vi "ROI entry screen-LBox edit cells.vi"(8 "error in (no error)":errorcluster, 11 "Selected Cell":T1) -> (0 "error out":errorcluster)   [LabVIEW 2020]
uses:
  <vilib>/Utility/miscctls.llb/LVRowAndColumnTypeDef.ctl
  Typedefs/ROI management FG states.ctl
  Typedefs/ROI Variable resolution info.ctl
  Typedefs/FGV ROI Time Ops.ctl
  Globals/gl_ROI Entry UI globals.vi
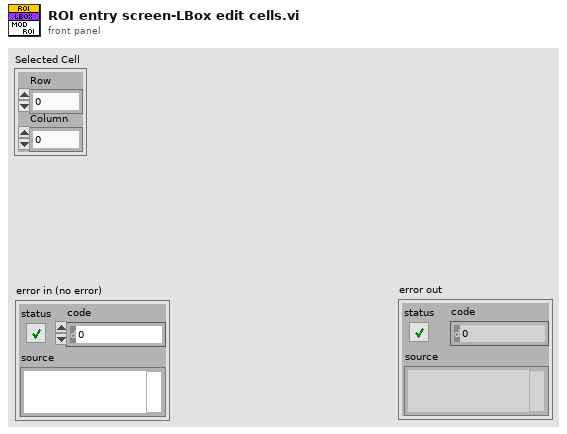
[diagram p1: front panel]
types:
  T1 = typedef "LVRowAndColumnTypeDef.ctl" = cluster{"Row":i32, "Column":i32}
  T2 = typedef "ROI management FG states.ctl" = enum16{"Read", "Write", "Write-from dataset", "Clear Last", "Clear All", "Delete ROI", "Update ROIs time", "Reload last ROI set", "Modify ROI Parameters", "Offset all ROI", "Offset visible ROI", "Modify Dwell Time", "Modify Laser Power"}
  T3 = typedef "ROI entry screen ctrl refs cluster.ctl" = cluster{"Done button":refnum<vi>, "Imaging button":refnum<vi>, "Acquisition button":refnum<vi>, "Scan dwell time per pixel (us)":refnum<vi>, "# of planes":refnum<vi>, "Zoom Ctrl":refnum<vi>, "Equal size":refnum<vi>, "Channel":refnum<vi>, "Image Display":refnum<vi>, "Z-Plane Selector":refnum<vi>, "Number of lines left":refnum<vi>, "Z-stack folder path":refnum<vi>, "POI Density":refnum<vi>, "Arb Plane Entry":refnum<vi>, "Whole Plane":refnum<vi>, "Line Mode":refnum<vi>, "Clear Last":refnum<vi>, "Clear All":refnum<vi>, "Delete Lines":refnum<vi>, "Trial Length (sec)":refnum<vi>, "Palette Type":refnum<vi>, "Intensity slider":refnum<vi>, "# POI":refnum<vi>, "Max Z Proj":refnum<vi>, "Zplane ind":refnum<vi>, "Wavelength (nm)":refnum<vi>, "Number of Trials":refnum<vi>, "Funct stim.trig.enable":refnum<vi>, "Funct stim.trig.delay (s)":refnum<vi>, "Line Mode":refnum<vi>, "Step size (µm)":refnum<vi>, "ROI move mode":refnum<vi>, "Cool-down time (s)":refnum<vi>, "Enable cool-down time":refnum<vi>, "Motor Z ind. (um)":refnum<vi>, "AOL Z ind. (um)":refnum<vi>, "Load Reference Image":refnum<vi>, "Rel.  Res.":refnum<vi>, "ROI LIST":refnum<vi>, "Show All":refnum<vi>, "ROI Type":refnum<vi>, "Start Plane":refnum<vi>, "Stop Plane":refnum<vi>, "Offset ROI":refnum<vi>, "Tab Control":refnum<vi>, "Laser Power(%)":refnum<vi>, "Cycle rate":refnum<vi>, "FOV (Ind.)":refnum<vi>, "Frame Size (Ind.)":refnum<vi>, "Resolution (Ind.)":refnum<vi>, "Pixel Density (Ind)":refnum<vi>, "Laser Power (Ind.)":refnum<vi>, "Dwell Time (Ind.)":refnum<vi>, "Adj MC":refnum<vi>}
  T4 = typedef "ROI parameters data type.ctl" = cluster{"ROI index":dbl, "ROI ID":dbl, "ROI Time (ns)":dbl, "Pixels in ROI":dbl, "X start":dbl, "Y start":dbl, "Z start":dbl, "X stop":dbl, "Y stop":dbl, "Z stop":dbl, "Angle (deg)":dbl, "Composite ID":dbl, "Number of lines":dbl, "Frame Size":dbl, "Zoom":dbl, "Laser Power (%)":dbl, "ROI group ID":dbl, "Resolution":dbl, "Dwell Time per pixel":dbl, "Pixels per miniscan":dbl, "Original FOV (um)":dbl, "Apparent Frame Size":dbl, "Z Plane Idx":i32[], "Z Plane codes":i32[]}
  T5 = typedef "ROI Variable resolution info.ctl" = cluster{"Resolution":dbl, "Pixel Density":dbl, "Relative Resolution":dbl, "Apparent frame size":dbl}
  T6 = typedef "FGV ROI Time Ops.ctl" = enum16{"Read", "Write Cycle Time", "Write Cycle Rate"}
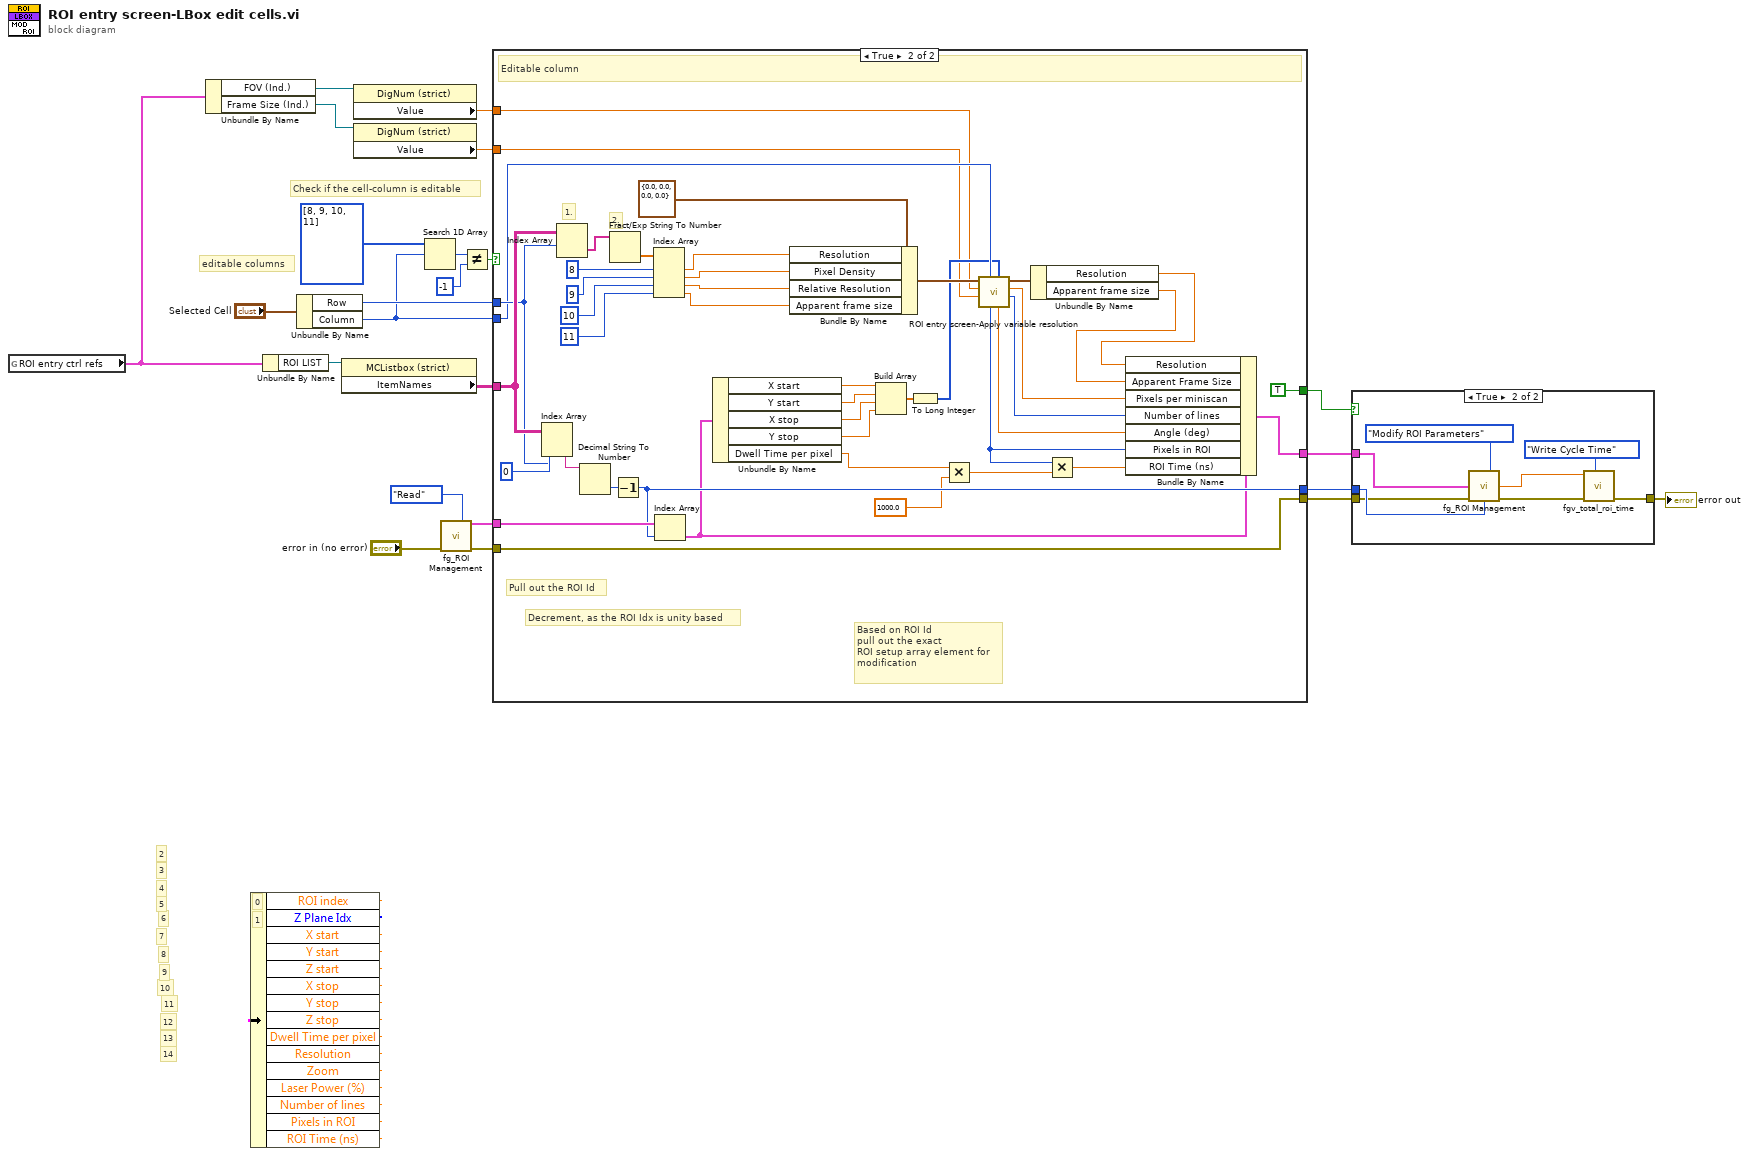
[diagram p0: block diagram]
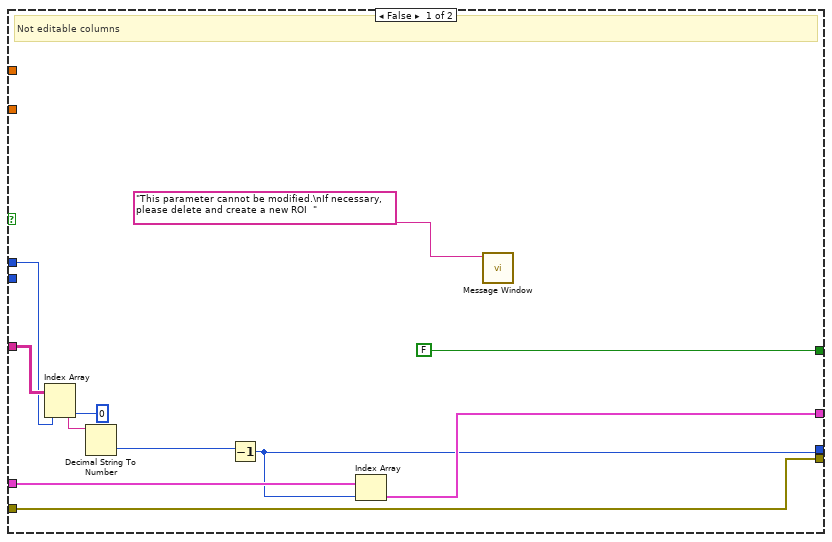
[diagram p3: hidden frame]
diagram:
  # "editable columns"
  # "Check if the cell-column is editable"
  # "14"
  # "13"
  # "12"
  # "11"
  # "10"
  # "9"
  # "8"
  # "7"
  # "6"
  # "5"
  # "4"
  # "3"
  # "2"
  # "1"
  # "0"
  n1 = global read "gl_ROI Entry UI globals.vi" "ROI entry ctrl refs"() -> (w3:T3)
  n2 = Unbundle By Name(w3) -> ("FOV (Ind.)"=w6:refnum<vi>, "Frame Size (Ind.)"=w5:refnum<vi>)
  n3 = Unbundle By Name(w3) -> ("ROI LIST"=w18:refnum<vi>)
  n4 = Unbundle By Name("Selected Cell") -> ("Row"=w16:i32, "Column"=w10:i32)
  n5 = property class="MCListbox (strict)"(reference=w18) -> ("ItemNames"=w17:string[][])  [unwired: 1 in, 2 out]
  n6 = property class="DigNum (strict)"(reference=w6) -> ("Value"=w2:dbl)  [unwired: 1 in, 2 out]
  n7 = property class="DigNum (strict)"(reference=w5) -> ("Value"=w1:dbl)  [unwired: 1 in, 2 out]
  n8 = Search 1D Array(1D array=i32[] [8, 9, 10, 11], element=w10) -> (index of element=w12:i32)  [unwired: 1 in]
  n9 = call "fg_ROI Management.vi"("Function"=ROI_management_FG_states."Read", "error in (no error)"="error in (no error)") -> ("ROI Setup"=w21:T4[], "error out"=w19:errorcluster)  [unwired: 7 in, 5 out]
  n10 = Not Equal?(x=w12, y=-1) -> (x != y?=w9:bool)
  n11 = case shown="True" w9 {
    tunnel: w21 -> [w29 w74]
    tunnel: [FALSE TRUE] -> w20
    tunnel: w19 -> [w25 w72]
    tunnel: w17 -> [w28 w71]
    tunnel: w16 -> [w27 w70]
    tunnel: [w26 w43] -> w15
    tunnel: [w24 w73] -> w14
    tunnel: w10 -> [_ w53]
    tunnel: [w25 w72] -> w8
    tunnel: w2 -> [_ w50]
    tunnel: w1 -> [_ w49]
    frame False {
      # "Not editable columns"
      n12 = Index Array(array=w28, index (row)=w27, index (col)=0 ("disabled index (col)")) -> (element=w31:string)
      n13 = Decimal String To Number(string=w31) -> (number=w30:i32)  [unwired: 2 in, 1 out]
      n14 = Decrement(x=w30) -> (x-1=w24:i32)
      n15 = Index Array(array=w29, index=w24) -> (element=w26:T4)
      n16 = call "Message Window.vi"("Message string"="This parameter cannot be modified.\nIf necessary, please delete and create a new ROI  ") -> ()  [unwired: 10 in, 1 out]
    }
    frame True {
      # "2."
      # "1."
      # "Decrement, as the ROI Idx is unity based"
      # "Based on ROI Id \npull out the exact\nROI setup array element for\nmodification"
      # "Pull out the ROI Id"
      # "Editable column"
      n17 = Index Array(array=w71, index (row)=w70, index (col)=0 ("disabled index (col)")) -> (element=w76:string)
      n18 = Index Array(array=w71, index (row)=w70) -> (element=w61:string[])  [unwired: 1 in]
      n19 = Decimal String To Number(string=w76) -> (number=w75:i32)  [unwired: 2 in, 1 out]
      n20 = Fract/Exp String To Number(string=w61) -> (number=w60:dbl[])  [unwired: 3 in, 1 out]
      n21 = Decrement(x=w75) -> (x-1=w73:i32)
      n22 = Index Array(array=w60, index #1=8 ("index"), index #2=9 ("index"), index #3=10 ("index"), index #4=11 ("index")) -> (element #1=w58:dbl, element #2=w57:dbl, element #3=w56:dbl, element #4=w55:dbl)
      n23 = Index Array(array=w74, index=w73) -> (element=w47:T4)
      n24 = Unbundle By Name(w47) -> ("X start"=w69:dbl, "Y start"=w68:dbl, "X stop"=w67:dbl, "Y stop"=w66:dbl, "Dwell Time per pixel"=w36:dbl)
      n25 = Bundle By Name(cluster=T5 {"Resolution"=0.0, "Pixel Density"=0.0, "Relative Resolution"=0.0, "Apparent frame size"=0.0} ("ROI Variable resolution info"), "Resolution"=w58, "Pixel Density"=w57, "Relative Resolution"=w56, "Apparent frame size"=w55) -> (w54:T5)
      n26 = Build Array(w69, w68, w67, w66) -> (w52:dbl[])
      n27 = To Long Integer(number=w52) -> (32bit integer=w51:i32[])
      n28 = Multiply(x=w36, y=1000.0) -> (x*y=w35:dbl)
      n29 = call "ROI entry screen-Apply variable resolution.vi"("XY Coordinates"=w51, "Changed column"=w53, "Frame Size (original)"=w49, "FOV (original)"=w50, "ROI Variable resolution info"=w54) -> ("No of lines in ROI"=w45:i32, "X pixels"=w46:dbl, "ROI Variable resolution info O/P"=w42:T5, "Angle (deg)"=w44:dbl, "Pixels in ROI"=w38:i32)  [unwired: 1 in, 1 out]
      n30 = Unbundle By Name(w42) -> ("Resolution"=w40:dbl, "Apparent frame size"=w41:dbl)
      n31 = Multiply(x=w38, y=w35) -> (x*y=w39:dbl)
      n32 = Bundle By Name(cluster=w47, "Resolution"=w40, "Apparent Frame Size"=w41, "Pixels per miniscan"=w46, "Number of lines"=w45, "Angle (deg)"=w44, "Pixels in ROI"=w38, "ROI Time (ns)"=w39) -> (w43:T4)
    }
  }
  n33 = case shown="True" w20 {
    tunnel: w15 -> [_ w85]
    tunnel: w14 -> [_ w84]
    tunnel: w8 -> [w78 w83]
    tunnel: [w78 w81] -> w7
    frame False {
    }
    frame True {
      n34 = call "fg_ROI Management.vi"("Function"=ROI_management_FG_states."Modify ROI Parameters", "XYZ"=w85, "error in (no error)"=w83, "ROI Setup Array Idx to modify"=w84) -> ("Total ROI time"=w80:dbl, "error out"=w82:errorcluster)  [unwired: 5 in, 5 out]
      n35 = call "fgv_total_roi_time.vi"("Op"=FGV_ROI_Time_Ops."Write Cycle Time", "error in (no error)"=w82, "Total cycle time"=w80) -> ("error out"=w81:errorcluster)  [unwired: 4 in, 4 out]
    }
  }
  "error out" <- w7
